vi "LSMcontroller_v59_PIzstage.vi"() -> ()   [LabVIEW 2015] (continued)
                    n4189 = call "tt_timeandsamples.vi"("bin"=w957, "refreshtime"=w951, "srateAODOtt"=w954, "tot#ofsamples"=w959) -> ("refreshrate"=w955:dbl, "refreshbuffer"=w956:i32, "timetracecycles"=w961:i32)  [unwired: 5 in]
                    n4190 = local read "bin"() -> (w958:dbl)
                    n4191 = call "2pparameters.vi"("command"="get") -> ("params out"=w970:T11)  [unwired: 1 in]
                    n4192 = Bundle By Name(cluster=w970, "Drawing Mode"=w943, "measpoints"=w959, "tt_cycles"=w961, "refreshbuffer"=w956, "refreshrate"=w955, "Vx-ref"=w962, "Vy-ref"=w964, "srate"=w953, "finite"=w966, "cont"=w965, "wavdet"=w967, "avpp"=w963, "srateAODO"=w960, "bufferAI"=w956, "bin"=w958, "Angle Img"=w950, "Vxminref"=w949, "Vxmaxref"=w948, "Vyminref"=w947, "Vymaxref"=w946, "Xpixels Img"=w945, "Ypixels Img"=w944, "Pel"=w942, "Vz-reset"=0.0, "AIoverride"=w940, "type"="Timetrace") -> (w968:T11)
                    n4193 = Reciprocal(x=w955) -> (1/x=w952:dbl)
                    n4194 = local write "refreshtime"(w952) -> ()
                    n4195 = call "2pparameters.vi"("Params in"=w968, "command"="set") -> ()  [unwired: 1 out]
                  }
                  frame "Lifetime (point)" {
                  }
                }
              }
              frame #1 {
                w973 = FALSE ("wavdet")
                n4196 = call "2pparameters.vi"("command"="get") -> ("params out"=w977:T11)  [unwired: 1 in]
                n4197 = Bundle By Name(cluster=w977, "finite"=w973, "cont"=w973, "wavdet"=TRUE) -> (w974:T11)
                n4198 = call "2pparameters.vi"("Params in"=w974, "command"="set") -> ()  [unwired: 1 out]
              }
              frame #2 {
                n4199 = local read "DO channels"() -> (w982:u16)
                n4200 = call "2pparameters.vi"("command"="get") -> ("params out"=w984:T11)  [unwired: 1 in]
                n4201 = Unbundle By Name(w984) -> ("aDO"=w983:u32[])
                n4202 = Search 1D Array(1D array=w983, element=w982) -> (index of element=w980:i32)  [unwired: 1 in]
                n4203 = Greater?(x=w980, y=-1) -> (0:w979:bool)
                n4204 = case shown="True" w979 {
                  tunnel: w980 -> [_ w993]
                  frame False {
                  }
                  frame True {
                    n4205 = local read "Meastab"() -> (w987:enum32{"X-Y Image", "Linescan", "Timetrace"})
                    n4206 = local read "Digital padding value"() -> (w988:dbl)
                    n4207 = local read "Digital time offset (s)"() -> (w989:dbl)
                    n4208 = case shown="\"Timetrace\"" w987 {
                      tunnel: [w994 w995] -> w986
                      frame "X-Y Image", Default {
                        n4209 = local read "Sampling rate"() -> (w994:dbl)
                      }
                      frame "Timetrace" {
                        n4210 = local read "srateAODOtt"() -> (w995:dbl)
                      }
                    }
                    n4211 = local read "Digital Freq (Hz)"() -> (w991:dbl)
                    n4212 = local read "Digital phase (s)"() -> (w990:dbl)
                    n4213 = local read "Digital DC (%)"() -> (w992:dbl)
                    n4214 = call "replace DO wf param.vi"("Digital Freq (Hz)"=w991, "Digital DC (%)"=w992, "Digital phase"=w990, "Sampling frequency (Hz)"=w986, "Digital time offset (s)"=w989, "index of DO wave"=w993, "padding value"=w988) -> ()  [unwired: 4 in]
                  }
                }
              }
              frame #3 {
                n4215 = case shown="True" w996 {
                  tunnel: w997 -> [_ w1004]
                  frame False {
                  }
                  frame True {
                    n4216 = local read "Meastab"() -> (w1001:enum32{"X-Y Image", "Linescan", "Timetrace"})
                    n4217 = call "waveformparamsv2.vi"("command"="get") -> ("Params out"=w1020:T15)  [unwired: 4 in, 2 out]
                    n4218 = Unbundle By Name(w1020) -> ("DO parameters"=w1019:T18)
                    n4219 = property on="refwf" class="Ring (strict)"() -> ("RingText.Text"=w1026:string)  [unwired: 2 in, 2 out]
                    n4220 = case shown="\"Timetrace\"" w1001 {
                      tunnel: [w1027 w1028] -> w1000
                      frame "X-Y Image", Default {
                        n4221 = local read "Sampling rate"() -> (w1027:dbl)
                      }
                      frame "Timetrace" {
                        n4222 = local read "srateAODOtt"() -> (w1028:dbl)
                      }
                    }
                    n4223 = call "waveformsAObuffer.vi"("command"="get") -> ("AO wf out"=w1024:waveform(dbl)[])  [unwired: 1 in]
                    n4224 = call "waveformsDObuffer.vi"("command"="get") -> ("DO wf out"=w1022:digitalwaveform[])  [unwired: 1 in]
                    n4225 = call "referfencesize.vi"("Digital waveforms in"=w1022, "Analog waveforms in"=w1024, "reference waveforms to"=w1026) -> ("number of samples"=w1017:i32)  [unwired: 2 in]
                    n4226 = Index Array(array=w1019, index=w1004) -> (element=w1018:T19)
                    n4227 = call "waveformsDObuffer.vi"("command"="get") -> ("DO wf out"=w1014:digitalwaveform[])  [unwired: 1 in]
                    n4228 = call "simple digital from wf params.vi"("waveform params"=w1018, "number of samples"=w1017) -> ("digital waveform"=w1016:digitalwaveform)
                    n4229 = property on="refwf" class="Ring (strict)"() -> ("RingText.Text"=w1006:string)  [unwired: 2 in, 2 out]
                    n4230 = Replace Array Subset(array=w1014, new element=w1016, index=w1004) -> (w1005:digitalwaveform[])
                    n4231 = call "waveformsAObuffer.vi"("command"="get") -> ("AO wf out"=w1013:waveform(dbl)[])  [unwired: 1 in]
                    n4232 = local read "wavdet"() -> (w1003:bool)
                    n4233 = call "correctwaveformsizetemp.vi"("new sampling frequency (Hz)"=w1000, "start"=FALSE, "reference waveforms to"=w1006, "Analog waveforms in"=w1013, "stop"=FALSE, "Digital waveforms in"=w1005) -> ("analog wf out"=w1009:waveform(dbl)[], "Digital wf out"=w1007:digitalwaveform[], "measpoints"=w1002:i32)
                    n4234 = local write "Analog Lines Plot"(w1009) -> ()
                    n4235 = call "GetNumCamFramesv2.vi"("Digital Waveform Graph"=w1007) -> ("Numeric"=w1008:i32)  [unwired: 10 in]
                    n4236 = local write "Digital Lines Plot"(w1007) -> ()
                    n4237 = case shown="True" w1003 {
                      tunnel: w1002 -> [_ w1029]
                      frame False {
                      }
                      frame True {
                        n4238 = local write "# of frames"(w1029) -> ()
                      }
                    }
                    n4239 = call "waveformsAObuffer.vi"("AO wf in"=w1009, "command"="set") -> ()  [unwired: 1 out]
                    n4240 = call "waveformsDObuffer.vi"("DO wf in"=w1007, "command"="set") -> ()  [unwired: 1 out]
                    n4241 = local write "Total Camera Frames"(w1008) -> ()
                  }
                }
              }
              frame #4 {
                n4242 = local read "finite samples"() -> (w1030:bool)
                n4243 = local read "continuous"() -> (w1031:bool)
                n4244 = local read "wavdet"() -> (w1032:bool)
                n4245 = call "2pparameters.vi"("command"="get") -> ("params out"=w1035:T11)  [unwired: 1 in]
                n4246 = Bundle By Name(cluster=w1035, "finite"=w1030, "cont"=w1031, "wavdet"=w1032) -> (w1033:T11)
                n4247 = call "2pparameters.vi"("Params in"=w1033, "command"="set") -> ()  [unwired: 1 out]
              }
            }
          }
          event "refwf": Value Change {
            n4248 = event-data() -> ()  [unwired: 1 in, 6 out]
            n4249 = stacked-sequence {
              frame #0 {
                n4250 = local read "Measurement"() -> (w1037:T4)
                n4251 = case shown="\"X-Y-t movie\", Default" w1037 {
                  frame "X-Y-t movie", Default {
                    n4252 = local read "avpp"() -> (w1058:i32)
                    n4253 = local read "Angle ref"() -> (w1057:dbl)
                    n4254 = local read "ROI Type"() -> (w1056:u16)
                    n4255 = local read "xpixels ref"() -> (w1053:i32)
                    n4256 = local read "Vx-min ref"() -> (w1052:dbl)
                    n4257 = local read "Vx-max ref"() -> (w1051:dbl)
                    n4258 = local read "ypixels ref"() -> (w1049:i32)
                    n4259 = local read "Vy-min ref"() -> (w1050:dbl)
                    n4260 = local read "Vy-max ref"() -> (w1046:dbl)
                    n4261 = local read "Sampling rate"() -> (w1040:dbl)
                    n4262 = local read "finite samples"() -> (w1041:bool)
                    n4263 = local read "continuous"() -> (w1044:bool)
                    n4264 = local read "wavdet"() -> (w1045:bool)
                    n4265 = local read "# of frames"() -> (w1043:i32)
                    n4266 = local read "maxbufferAI"() -> (w1042:i32)
                    n4267 = local read "Override AI buffer"() -> (w1038:bool)
                    n4268 = call "2pparameters.vi"("command"="get") -> ("params out"=w1055:T11)  [unwired: 1 in]
                    n4269 = Bundle By Name(cluster=w1055, "type"="X-Y-t movie", "avpp"=w1058, "Angle Img"=w1057, "Xpixels Img"=w1053, "Vx-min Img"=w1052, "VX-max Img"=w1051, "Ypixels Img"=w1049, "Vy-min Img"=w1050, "Vy-max Img"=w1046, "srate"=w1040, "srate Img"=w1040, "finite"=w1041, "cont"=w1044, "wavdet"=w1045, "measpoints"=w1043, "maxbufferAI"=w1042, "Drawing Mode"=w1056, "Vz-reset"=0.0, "AIoverride"=w1038) -> (w1047:T11)
                    n4270 = call "2pparameters.vi"("Params in"=w1047, "command"="set") -> ()  [unwired: 1 out]
                  }
                  frame "X-Y-Z stack" {
                    n4271 = call "2pparameters.vi"("command"="get") -> ("params out"=w1062:T11)  [unwired: 1 in]
                    n4272 = Bundle By Name(cluster=w1062, "type"="X-Y-Z stack") -> (w1060:T11)
                    n4273 = call "2pparameters.vi"("Params in"=w1060, "command"="set") -> ()  [unwired: 1 out]
                  }
                  frame "Lifetime (scan)" {
                    n4274 = call "2pparameters.vi"("command"="get") -> ("params out"=w1067:T11)  [unwired: 1 in]
                    n4275 = Bundle By Name(cluster=w1067, "type"="Lifetime (scan)") -> (w1065:T11)
                    n4276 = call "2pparameters.vi"("Params in"=w1065, "command"="set") -> ()  [unwired: 1 out]
                  }
                  frame "Lifetime (contour)" {
                    n4277 = local read "Vy-min draw"() -> (w1077:dbl)
                    n4278 = local read "Vy-max draw"() -> (w1076:dbl)
                    n4279 = local read "Vx-min draw"() -> (w1079:dbl)
                    n4280 = local read "Vx-max draw"() -> (w1078:dbl)
                    n4281 = local read "xpixels ref"() -> (w1075:i32)
                    n4282 = local read "ypixels ref"() -> (w1074:i32)
                    n4283 = local read "ROI Type"() -> (w1073:u16)
                    n4284 = local read "srateAODOtt"() -> (w1084:dbl)
                    n4285 = local read "# of frames"() -> (w1089:i32)
                    n4286 = local read "refreshtime"() -> (w1081:dbl)
                    n4287 = local read "Pel"() -> (w1072:dbl)
                    n4288 = local read "bin"() -> (w1087:dbl)
                    n4289 = local read "Override AI buffer"() -> (w1070:bool)
                    n4290 = local read "finite samples"() -> (w1096:bool)
                    n4291 = local read "srateAODOtt"() -> (w1083:dbl)
                    n4292 = local read "srateAODOtt"() -> (w1090:dbl)
                    n4293 = local read "continuous"() -> (w1095:bool)
                    n4294 = local read "Angle ref"() -> (w1080:dbl)
                    n4295 = local read "wavdet"() -> (w1097:bool)
                    n4296 = local read "Vx-ref"() -> (w1092:dbl)
                    n4297 = local read "Vy-ref"() -> (w1094:dbl)
                    n4298 = local read "avpp"() -> (w1093:i32)
                    n4299 = call "tt_timeandsamples.vi"("bin"=w1087, "refreshtime"=w1081, "srateAODOtt"=w1084, "tot#ofsamples"=w1089) -> ("refreshrate"=w1085:dbl, "refreshbuffer"=w1086:i32, "timetracecycles"=w1091:i32)  [unwired: 5 in]
                    n4300 = local read "bin"() -> (w1088:dbl)
                    n4301 = call "2pparameters.vi"("command"="get") -> ("params out"=w1100:T11)  [unwired: 1 in]
                    n4302 = Bundle By Name(cluster=w1100, "Drawing Mode"=w1073, "measpoints"=w1089, "tt_cycles"=w1091, "refreshbuffer"=w1086, "refreshrate"=w1085, "Vx-ref"=w1092, "Vy-ref"=w1094, "srate"=w1083, "finite"=w1096, "cont"=w1095, "wavdet"=w1097, "avpp"=w1093, "srateAODO"=w1090, "bufferAI"=w1086, "bin"=w1088, "Angle Img"=w1080, "Vxminref"=w1079, "Vxmaxref"=w1078, "Vyminref"=w1077, "Vymaxref"=w1076, "Xpixels Img"=w1075, "Ypixels Img"=w1074, "Pel"=w1072, "Vz-reset"=0.0, "AIoverride"=w1070, "type"="Lifetime (contour)") -> (w1098:T11)
                    n4303 = Reciprocal(x=w1085) -> (1/x=w1082:dbl)
                    n4304 = local write "refreshtime"(w1082) -> ()
                    n4305 = call "2pparameters.vi"("Params in"=w1098, "command"="set") -> ()  [unwired: 1 out]
                  }
                  frame "X-Y-Z-t movie" {
                  }
                  frame "linescan" {
                  }
                  frame "Timetrace" {
                    n4306 = local read "Vy-min draw"() -> (w1110:dbl)
                    n4307 = local read "Vy-max draw"() -> (w1109:dbl)
                    n4308 = local read "Vx-min draw"() -> (w1112:dbl)
                    n4309 = local read "Vx-max draw"() -> (w1111:dbl)
                    n4310 = local read "xpixels ref"() -> (w1108:i32)
                    n4311 = local read "ypixels ref"() -> (w1107:i32)
                    n4312 = local read "ROI Type"() -> (w1106:u16)
                    n4313 = local read "srateAODOtt"() -> (w1117:dbl)
                    n4314 = local read "# of frames"() -> (w1122:i32)
                    n4315 = local read "refreshtime"() -> (w1114:dbl)
                    n4316 = local read "Pel"() -> (w1105:dbl)
                    n4317 = local read "bin"() -> (w1120:dbl)
                    n4318 = local read "Override AI buffer"() -> (w1103:bool)
                    n4319 = local read "finite samples"() -> (w1129:bool)
                    n4320 = local read "srateAODOtt"() -> (w1116:dbl)
                    n4321 = local read "srateAODOtt"() -> (w1123:dbl)
                    n4322 = local read "continuous"() -> (w1128:bool)
                    n4323 = local read "Angle ref"() -> (w1113:dbl)
                    n4324 = local read "wavdet"() -> (w1130:bool)
                    n4325 = local read "Vx-ref"() -> (w1125:dbl)
                    n4326 = local read "Vy-ref"() -> (w1127:dbl)
                    n4327 = local read "avpp"() -> (w1126:i32)
                    n4328 = call "tt_timeandsamples.vi"("bin"=w1120, "refreshtime"=w1114, "srateAODOtt"=w1117, "tot#ofsamples"=w1122) -> ("refreshrate"=w1118:dbl, "refreshbuffer"=w1119:i32, "timetracecycles"=w1124:i32)  [unwired: 5 in]
                    n4329 = local read "bin"() -> (w1121:dbl)
                    n4330 = call "2pparameters.vi"("command"="get") -> ("params out"=w1133:T11)  [unwired: 1 in]
                    n4331 = Bundle By Name(cluster=w1133, "Drawing Mode"=w1106, "measpoints"=w1122, "tt_cycles"=w1124, "refreshbuffer"=w1119, "refreshrate"=w1118, "Vx-ref"=w1125, "Vy-ref"=w1127, "srate"=w1116, "finite"=w1129, "cont"=w1128, "wavdet"=w1130, "avpp"=w1126, "srateAODO"=w1123, "bufferAI"=w1119, "bin"=w1121, "Angle Img"=w1113, "Vxminref"=w1112, "Vxmaxref"=w1111, "Vyminref"=w1110, "Vymaxref"=w1109, "Xpixels Img"=w1108, "Ypixels Img"=w1107, "Pel"=w1105, "Vz-reset"=0.0, "AIoverride"=w1103, "type"="Timetrace") -> (w1131:T11)
                    n4332 = Reciprocal(x=w1118) -> (1/x=w1115:dbl)
                    n4333 = local write "refreshtime"(w1115) -> ()
                    n4334 = call "2pparameters.vi"("Params in"=w1131, "command"="set") -> ()  [unwired: 1 out]
                  }
                  frame "Lifetime (point)" {
                  }
                }
              }
              frame #1 {
                w1136 = FALSE ("wavdet")
                n4335 = call "2pparameters.vi"("command"="get") -> ("params out"=w1140:T11)  [unwired: 1 in]
                n4336 = Bundle By Name(cluster=w1140, "finite"=w1136, "cont"=w1136, "wavdet"=TRUE) -> (w1137:T11)
                n4337 = call "2pparameters.vi"("Params in"=w1137, "command"="set") -> ()  [unwired: 1 out]
              }
              frame #2 {
                n4338 = local read "Meastab"() -> (w1145:enum32{"X-Y Image", "Linescan", "Timetrace"})
                n4339 = property on="refwf" class="Ring (strict)"() -> ("RingText.Text"=w1148:string)  [unwired: 2 in, 2 out]
                n4340 = case shown="\"Timetrace\"" w1145 {
                  tunnel: [w1158 w1159] -> w1144
                  frame "X-Y Image", Default {
                    n4341 = local read "Sampling rate"() -> (w1158:dbl)
                  }
                  frame "Timetrace" {
                    n4342 = local read "srateAODOtt"() -> (w1159:dbl)
                  }
                }
                n4343 = call "waveformsAObuffer.vi"("command"="get") -> ("AO wf out"=w1157:waveform(dbl)[])  [unwired: 1 in]
                n4344 = local read "wavdet"() -> (w1147:bool)
                n4345 = call "waveformsDObuffer.vi"("command"="get") -> ("DO wf out"=w1153:digitalwaveform[])  [unwired: 1 in]
                n4346 = call "correctwaveformsizetemp.vi"("new sampling frequency (Hz)"=w1144, "start"=FALSE, "reference waveforms to"=w1148, "Analog waveforms in"=w1157, "stop"=FALSE, "Digital waveforms in"=w1153) -> ("analog wf out"=w1151:waveform(dbl)[], "Digital wf out"=w1149:digitalwaveform[], "measpoints"=w1146:i32)
                n4347 = local write "Analog Lines Plot"(w1151) -> ()
                n4348 = call "GetNumCamFramesv2.vi"("Digital Waveform Graph"=w1149) -> ("Numeric"=w1150:i32)  [unwired: 10 in]
                n4349 = local write "Digital Lines Plot"(w1149) -> ()
                n4350 = call "waveformsDObuffer.vi"("DO wf in"=w1149, "command"="set") -> ()  [unwired: 1 out]
                n4351 = call "waveformsAObuffer.vi"("AO wf in"=w1151, "command"="set") -> ()  [unwired: 1 out]
                n4352 = local write "Total Camera Frames"(w1150) -> ()
                n4353 = case shown="True" w1147 {
                  tunnel: w1146 -> [_ w1160]
                  frame False {
                  }
                  frame True {
                    n4354 = local write "# of frames"(w1160) -> ()
                  }
                }
              }
              frame #3 {
                n4355 = local read "finite samples"() -> (w1161:bool)
                n4356 = local read "continuous"() -> (w1162:bool)
                n4357 = local read "wavdet"() -> (w1163:bool)
                n4358 = call "2pparameters.vi"("command"="get") -> ("params out"=w1166:T11)  [unwired: 1 in]
                n4359 = Bundle By Name(cluster=w1166, "finite"=w1161, "cont"=w1162, "wavdet"=w1163) -> (w1164:T11)
                n4360 = call "2pparameters.vi"("Params in"=w1164, "command"="set") -> ()  [unwired: 1 out]
              }
            }
          }
          event "Start amplitude (V)", "Cycles", "Baseline (V)", "Step size (V)", "DC (%)", "Period (ms)", "Repeats", "Pulses", "phase shift (ms)": Value Change {
            n4361 = event-data() -> ()  [unwired: 1 in, 6 out]
            n4362 = stacked-sequence {
              seq-local: [_ _ w1274 _ _] -> [_ _ _ w1296 _]
              seq-local: [_ _ w1273 _ _] -> [_ _ _ w1295 _]
              frame #0 {
                n4363 = local read "Measurement"() -> (w1168:T4)
                n4364 = case shown="\"X-Y-t movie\", Default" w1168 {
                  frame "X-Y-t movie", Default {
                    n4365 = local read "avpp"() -> (w1189:i32)
                    n4366 = local read "Angle ref"() -> (w1188:dbl)
                    n4367 = local read "ROI Type"() -> (w1187:u16)
                    n4368 = local read "xpixels ref"() -> (w1184:i32)
                    n4369 = local read "Vx-min ref"() -> (w1183:dbl)
                    n4370 = local read "Vx-max ref"() -> (w1182:dbl)
                    n4371 = local read "ypixels ref"() -> (w1180:i32)
                    n4372 = local read "Vy-min ref"() -> (w1181:dbl)
                    n4373 = local read "Vy-max ref"() -> (w1177:dbl)
                    n4374 = local read "Sampling rate"() -> (w1171:dbl)
                    n4375 = local read "finite samples"() -> (w1172:bool)
                    n4376 = local read "continuous"() -> (w1175:bool)
                    n4377 = local read "wavdet"() -> (w1176:bool)
                    n4378 = local read "# of frames"() -> (w1174:i32)
                    n4379 = local read "maxbufferAI"() -> (w1173:i32)
                    n4380 = local read "Override AI buffer"() -> (w1169:bool)
                    n4381 = call "2pparameters.vi"("command"="get") -> ("params out"=w1186:T11)  [unwired: 1 in]
                    n4382 = Bundle By Name(cluster=w1186, "type"="X-Y-t movie", "avpp"=w1189, "Angle Img"=w1188, "Xpixels Img"=w1184, "Vx-min Img"=w1183, "VX-max Img"=w1182, "Ypixels Img"=w1180, "Vy-min Img"=w1181, "Vy-max Img"=w1177, "srate"=w1171, "srate Img"=w1171, "finite"=w1172, "cont"=w1175, "wavdet"=w1176, "measpoints"=w1174, "maxbufferAI"=w1173, "Drawing Mode"=w1187, "Vz-reset"=0.0, "AIoverride"=w1169) -> (w1178:T11)
                    n4383 = call "2pparameters.vi"("Params in"=w1178, "command"="set") -> ()  [unwired: 1 out]
                  }
                  frame "X-Y-Z stack" {
                    n4384 = call "2pparameters.vi"("command"="get") -> ("params out"=w1193:T11)  [unwired: 1 in]
                    n4385 = Bundle By Name(cluster=w1193, "type"="X-Y-Z stack") -> (w1191:T11)
                    n4386 = call "2pparameters.vi"("Params in"=w1191, "command"="set") -> ()  [unwired: 1 out]
                  }
                  frame "Lifetime (scan)" {
                    n4387 = call "2pparameters.vi"("command"="get") -> ("params out"=w1198:T11)  [unwired: 1 in]
                    n4388 = Bundle By Name(cluster=w1198, "type"="Lifetime (scan)") -> (w1196:T11)
                    n4389 = call "2pparameters.vi"("Params in"=w1196, "command"="set") -> ()  [unwired: 1 out]
                  }
                  frame "Lifetime (contour)" {
                    n4390 = local read "Vy-min draw"() -> (w1208:dbl)
                    n4391 = local read "Vy-max draw"() -> (w1207:dbl)
                    n4392 = local read "Vx-min draw"() -> (w1210:dbl)
                    n4393 = local read "Vx-max draw"() -> (w1209:dbl)
                    n4394 = local read "xpixels ref"() -> (w1206:i32)
                    n4395 = local read "ypixels ref"() -> (w1205:i32)
                    n4396 = local read "ROI Type"() -> (w1204:u16)
                    n4397 = local read "srateAODOtt"() -> (w1215:dbl)
                    n4398 = local read "# of frames"() -> (w1220:i32)
                    n4399 = local read "refreshtime"() -> (w1212:dbl)
                    n4400 = local read "Pel"() -> (w1203:dbl)
                    n4401 = local read "bin"() -> (w1218:dbl)
                    n4402 = local read "Override AI buffer"() -> (w1201:bool)
                    n4403 = local read "finite samples"() -> (w1227:bool)
                    n4404 = local read "srateAODOtt"() -> (w1214:dbl)
                    n4405 = local read "srateAODOtt"() -> (w1221:dbl)
                    n4406 = local read "continuous"() -> (w1226:bool)
                    n4407 = local read "Angle ref"() -> (w1211:dbl)
                    n4408 = local read "wavdet"() -> (w1228:bool)
                    n4409 = local read "Vx-ref"() -> (w1223:dbl)
                    n4410 = local read "Vy-ref"() -> (w1225:dbl)
                    n4411 = local read "avpp"() -> (w1224:i32)
                    n4412 = call "tt_timeandsamples.vi"("bin"=w1218, "refreshtime"=w1212, "srateAODOtt"=w1215, "tot#ofsamples"=w1220) -> ("refreshrate"=w1216:dbl, "refreshbuffer"=w1217:i32, "timetracecycles"=w1222:i32)  [unwired: 5 in]
                    n4413 = local read "bin"() -> (w1219:dbl)
                    n4414 = call "2pparameters.vi"("command"="get") -> ("params out"=w1231:T11)  [unwired: 1 in]
                    n4415 = Bundle By Name(cluster=w1231, "Drawing Mode"=w1204, "measpoints"=w1220, "tt_cycles"=w1222, "refreshbuffer"=w1217, "refreshrate"=w1216, "Vx-ref"=w1223, "Vy-ref"=w1225, "srate"=w1214, "finite"=w1227, "cont"=w1226, "wavdet"=w1228, "avpp"=w1224, "srateAODO"=w1221, "bufferAI"=w1217, "bin"=w1219, "Angle Img"=w1211, "Vxminref"=w1210, "Vxmaxref"=w1209, "Vyminref"=w1208, "Vymaxref"=w1207, "Xpixels Img"=w1206, "Ypixels Img"=w1205, "Pel"=w1203, "Vz-reset"=0.0, "AIoverride"=w1201, "type"="Lifetime (contour)") -> (w1229:T11)
                    n4416 = Reciprocal(x=w1216) -> (1/x=w1213:dbl)
                    n4417 = local write "refreshtime"(w1213) -> ()
                    n4418 = call "2pparameters.vi"("Params in"=w1229, "command"="set") -> ()  [unwired: 1 out]
                  }
                  frame "X-Y-Z-t movie" {
                  }
                  frame "linescan" {
                  }
                  frame "Timetrace" {
                    n4419 = local read "Vy-min draw"() -> (w1241:dbl)
                    n4420 = local read "Vy-max draw"() -> (w1240:dbl)
                    n4421 = local read "Vx-min draw"() -> (w1243:dbl)
                    n4422 = local read "Vx-max draw"() -> (w1242:dbl)
                    n4423 = local read "xpixels ref"() -> (w1239:i32)
                    n4424 = local read "ypixels ref"() -> (w1238:i32)
                    n4425 = local read "ROI Type"() -> (w1237:u16)
                    n4426 = local read "srateAODOtt"() -> (w1248:dbl)
                    n4427 = local read "# of frames"() -> (w1253:i32)
                    n4428 = local read "refreshtime"() -> (w1245:dbl)
                    n4429 = local read "Pel"() -> (w1236:dbl)
                    n4430 = local read "bin"() -> (w1251:dbl)
                    n4431 = local read "Override AI buffer"() -> (w1234:bool)
                    n4432 = local read "finite samples"() -> (w1260:bool)
                    n4433 = local read "srateAODOtt"() -> (w1247:dbl)
                    n4434 = local read "srateAODOtt"() -> (w1254:dbl)
                    n4435 = local read "continuous"() -> (w1259:bool)
                    n4436 = local read "Angle ref"() -> (w1244:dbl)
                    n4437 = local read "wavdet"() -> (w1261:bool)
                    n4438 = local read "Vx-ref"() -> (w1256:dbl)
                    n4439 = local read "Vy-ref"() -> (w1258:dbl)
                    n4440 = local read "avpp"() -> (w1257:i32)
                    n4441 = call "tt_timeandsamples.vi"("bin"=w1251, "refreshtime"=w1245, "srateAODOtt"=w1248, "tot#ofsamples"=w1253) -> ("refreshrate"=w1249:dbl, "refreshbuffer"=w1250:i32, "timetracecycles"=w1255:i32)  [unwired: 5 in]
                    n4442 = local read "bin"() -> (w1252:dbl)
                    n4443 = call "2pparameters.vi"("command"="get") -> ("params out"=w1264:T11)  [unwired: 1 in]
                    n4444 = Bundle By Name(cluster=w1264, "Drawing Mode"=w1237, "measpoints"=w1253, "tt_cycles"=w1255, "refreshbuffer"=w1250, "refreshrate"=w1249, "Vx-ref"=w1256, "Vy-ref"=w1258, "srate"=w1247, "finite"=w1260, "cont"=w1259, "wavdet"=w1261, "avpp"=w1257, "srateAODO"=w1254, "bufferAI"=w1250, "bin"=w1252, "Angle Img"=w1244, "Vxminref"=w1243, "Vxmaxref"=w1242, "Vyminref"=w1241, "Vymaxref"=w1240, "Xpixels Img"=w1239, "Ypixels Img"=w1238, "Pel"=w1236, "Vz-reset"=0.0, "AIoverride"=w1234, "type"="Timetrace") -> (w1262:T11)
                    n4445 = Reciprocal(x=w1249) -> (1/x=w1246:dbl)
                    n4446 = local write "refreshtime"(w1246) -> ()
                    n4447 = call "2pparameters.vi"("Params in"=w1262, "command"="set") -> ()  [unwired: 1 out]
                  }
                  frame "Lifetime (point)" {
                  }
                }
              }
              frame #1 {
                w1267 = FALSE ("wavdet")
                n4448 = call "2pparameters.vi"("command"="get") -> ("params out"=w1271:T11)  [unwired: 1 in]
                n4449 = Bundle By Name(cluster=w1271, "finite"=w1267, "cont"=w1267, "wavdet"=TRUE) -> (w1268:T11)
                n4450 = call "2pparameters.vi"("Params in"=w1268, "command"="set") -> ()  [unwired: 1 out]
              }
              frame #2 {
                n4451 = local read "AO channels"() -> (w1276:u32)
                n4452 = call "2pparameters.vi"("command"="get") -> ("params out"=w1278:T11)  [unwired: 1 in]
                n4453 = Unbundle By Name(w1278) -> ("aAO"=w1277:u32[])
                n4454 = Search 1D Array(1D array=w1277, element=w1276) -> (index of element=w1274:i32)  [unwired: 1 in]
                n4455 = Greater?(x=w1274, y=-1) -> (0:w1273:bool)
                n4456 = case shown="True" w1273 {
                  tunnel: w1274 -> [_ w1292]
                  frame False {
                  }
                  frame True {
                    n4457 = local read "Meastab"() -> (w1281:enum32{"X-Y Image", "Linescan", "Timetrace"})
                    n4458 = case shown="\"Timetrace\"" w1281 {
                      tunnel: [w1293 w1294] -> w1280
                      frame "X-Y Image", Default {
                        n4459 = local read "Sampling rate"() -> (w1293:dbl)
                      }
                      frame "Timetrace" {
                        n4460 = local read "srateAODOtt"() -> (w1294:dbl)
                      }
                    }
                    n4461 = local read "Start amplitude (V)"() -> (w1289:dbl)
                    n4462 = local read "phase shift (ms)"() -> (w1284:dbl)
                    n4463 = local read "Step size (V)"() -> (w1287:dbl)
                    n4464 = local read "Baseline (V)"() -> (w1288:dbl)
                    n4465 = local read "Period (ms)"() -> (w1285:dbl)
                    n4466 = local read "padding value"() -> (w1282:dbl)
                    n4467 = local read "Repeats"() -> (w1291:dbl)
                    n4468 = local read "Cycles"() -> (w1290:dbl)
                    n4469 = local read "DC (%)"() -> (w1286:dbl)
                    n4470 = local read "Pulses"() -> (w1283:dbl)
                    n4471 = call "replace AO square wf param.vi"("Baseline (V)"=w1288, "Start amplitude (V)"=w1289, "Cycles"=w1290, "Repeats"=w1291, "index of AO wave"=w1292, "Step size (V)"=w1287, "DC (%)"=w1286, "Sampling frequency (Hz)"=w1280, "Period (ms)"=w1285, "Cycle length (s)"=w1284, "Pulses"=w1283, "padding value"=w1282) -> ()  [unwired: 4 in]
                  }
                }
              }
              frame #3 {
                n4472 = case shown="True" w1295 {
                  tunnel: w1296 -> [_ w1304]
                  frame False {
                  }
                  frame True {
                    n4473 = call "waveformparamsv2.vi"("command"="get") -> ("Params out"=w1318:T15)  [unwired: 4 in, 2 out]
                    n4474 = Unbundle By Name(w1318) -> ("AO parameters"=w1317:T16)
                    n4475 = local read "Meastab"() -> (w1299:enum32{"X-Y Image", "Linescan", "Timetrace"})
                    n4476 = case shown="\"Timetrace\"" w1299 {
                      tunnel: [w1320 w1321] -> w1308
                      frame "X-Y Image", Default {
                        n4477 = local read "Sampling rate"() -> (w1320:dbl)
                      }
                      frame "Timetrace" {
                        n4478 = local read "srateAODOtt"() -> (w1321:dbl)
                      }
                    }
                    n4479 = Index Array(array=w1317, index=w1304) -> (element=w1306:T17)
                    n4480 = call "waveformsAObuffer.vi"("command"="get") -> ("AO wf out"=w1305:waveform(dbl)[])  [unwired: 1 in]
                    n4481 = call "generateRampedSquareWave_fromAOparameters.vi"("AO params"=w1306) -> ("Waveform"=w1303:waveform(dbl))  [unwired: 1 out]
                    n4482 = property on="refwf" class="Ring (strict)"() -> ("RingText.Text"=w1307:string)  [unwired: 2 in, 2 out]
                    n4483 = Replace Array Subset(array=w1305, new element=w1303, index=w1304) -> (w1302:waveform(dbl)[])
                    n4484 = call "waveformsDObuffer.vi"("command"="get") -> ("DO wf out"=w1313:digitalwaveform[])  [unwired: 1 in]
                    n4485 = call "correctwaveformsizetemp.vi"("new sampling frequency (Hz)"=w1308, "start"=FALSE, "reference waveforms to"=w1307, "Analog waveforms in"=w1302, "stop"=FALSE, "Digital waveforms in"=w1313) -> ("analog wf out"=w1311:waveform(dbl)[], "Digital wf out"=w1309:digitalwaveform[], "measpoints"=w1300:i32)
                    n4486 = local read "wavdet"() -> (w1301:bool)
                    n4487 = local write "Analog Lines Plot"(w1311) -> ()
                    n4488 = call "GetNumCamFramesv2.vi"("Digital Waveform Graph"=w1309) -> ("Numeric"=w1310:i32)  [unwired: 10 in]
                    n4489 = local write "Digital Lines Plot"(w1309) -> ()
                    n4490 = call "waveformsAObuffer.vi"("AO wf in"=w1311, "command"="set") -> ()  [unwired: 1 out]
                    n4491 = call "waveformsDObuffer.vi"("DO wf in"=w1309, "command"="set") -> ()  [unwired: 1 out]
                    n4492 = local write "Total Camera Frames"(w1310) -> ()
                    n4493 = case shown="True" w1301 {
                      tunnel: w1300 -> [_ w1322]
                      frame False {
                      }
                      frame True {
                        n4494 = local write "# of frames"(w1322) -> ()
                      }
                    }
                  }
                }
              }
              frame #4 {
                n4495 = local read "finite samples"() -> (w1323:bool)
                n4496 = local read "continuous"() -> (w1324:bool)
                n4497 = local read "wavdet"() -> (w1325:bool)
                n4498 = call "2pparameters.vi"("command"="get") -> ("params out"=w1328:T11)  [unwired: 1 in]
                n4499 = Bundle By Name(cluster=w1328, "finite"=w1323, "cont"=w1324, "wavdet"=w1325) -> (w1326:T11)
                n4500 = call "2pparameters.vi"("Params in"=w1326, "command"="set") -> ()  [unwired: 1 out]
              }
            }
          }
          event "Amplitude (V)", "Offset (V)", "Frequency", "Tri Repeats": Value Change {
            n4501 = event-data() -> ()  [unwired: 1 in, 6 out]
            n4502 = stacked-sequence {
              seq-local: [_ _ w1436 _ _] -> [_ _ _ w1454 _]
              seq-local: [_ _ w1435 _ _] -> [_ _ _ w1453 _]
              frame #0 {
                n4503 = local read "Measurement"() -> (w1330:T4)
                n4504 = case shown="\"X-Y-t movie\", Default" w1330 {
                  frame "X-Y-t movie", Default {
                    n4505 = local read "avpp"() -> (w1351:i32)
                    n4506 = local read "Angle ref"() -> (w1350:dbl)
                    n4507 = local read "ROI Type"() -> (w1349:u16)
                    n4508 = local read "xpixels ref"() -> (w1346:i32)
                    n4509 = local read "Vx-min ref"() -> (w1345:dbl)
                    n4510 = local read "Vx-max ref"() -> (w1344:dbl)
                    n4511 = local read "ypixels ref"() -> (w1342:i32)
                    n4512 = local read "Vy-min ref"() -> (w1343:dbl)
                    n4513 = local read "Vy-max ref"() -> (w1339:dbl)
                    n4514 = local read "Sampling rate"() -> (w1333:dbl)
                    n4515 = local read "finite samples"() -> (w1334:bool)
                    n4516 = local read "continuous"() -> (w1337:bool)
                    n4517 = local read "wavdet"() -> (w1338:bool)
                    n4518 = local read "# of frames"() -> (w1336:i32)
                    n4519 = local read "maxbufferAI"() -> (w1335:i32)
                    n4520 = local read "Override AI buffer"() -> (w1331:bool)
                    n4521 = call "2pparameters.vi"("command"="get") -> ("params out"=w1348:T11)  [unwired: 1 in]
                    n4522 = Bundle By Name(cluster=w1348, "type"="X-Y-t movie", "avpp"=w1351, "Angle Img"=w1350, "Xpixels Img"=w1346, "Vx-min Img"=w1345, "VX-max Img"=w1344, "Ypixels Img"=w1342, "Vy-min Img"=w1343, "Vy-max Img"=w1339, "srate"=w1333, "srate Img"=w1333, "finite"=w1334, "cont"=w1337, "wavdet"=w1338, "measpoints"=w1336, "maxbufferAI"=w1335, "Drawing Mode"=w1349, "Vz-reset"=0.0, "AIoverride"=w1331) -> (w1340:T11)
                    n4523 = call "2pparameters.vi"("Params in"=w1340, "command"="set") -> ()  [unwired: 1 out]
                  }
                  frame "X-Y-Z stack" {
                    n4524 = call "2pparameters.vi"("command"="get") -> ("params out"=w1355:T11)  [unwired: 1 in]
                    n4525 = Bundle By Name(cluster=w1355, "type"="X-Y-Z stack") -> (w1353:T11)
                    n4526 = call "2pparameters.vi"("Params in"=w1353, "command"="set") -> ()  [unwired: 1 out]
                  }
                  frame "Lifetime (scan)" {
                    n4527 = call "2pparameters.vi"("command"="get") -> ("params out"=w1360:T11)  [unwired: 1 in]
                    n4528 = Bundle By Name(cluster=w1360, "type"="Lifetime (scan)") -> (w1358:T11)
                    n4529 = call "2pparameters.vi"("Params in"=w1358, "command"="set") -> ()  [unwired: 1 out]
                  }
                  frame "Lifetime (contour)" {
                    n4530 = local read "Vy-min draw"() -> (w1370:dbl)
                    n4531 = local read "Vy-max draw"() -> (w1369:dbl)
                    n4532 = local read "Vx-min draw"() -> (w1372:dbl)
                    n4533 = local read "Vx-max draw"() -> (w1371:dbl)
                    n4534 = local read "xpixels ref"() -> (w1368:i32)
                    n4535 = local read "ypixels ref"() -> (w1367:i32)
                    n4536 = local read "ROI Type"() -> (w1366:u16)
                    n4537 = local read "srateAODOtt"() -> (w1377:dbl)
                    n4538 = local read "# of frames"() -> (w1382:i32)
                    n4539 = local read "refreshtime"() -> (w1374:dbl)
                    n4540 = local read "Pel"() -> (w1365:dbl)
                    n4541 = local read "bin"() -> (w1380:dbl)
                    n4542 = local read "Override AI buffer"() -> (w1363:bool)
                    n4543 = local read "finite samples"() -> (w1389:bool)
                    n4544 = local read "srateAODOtt"() -> (w1376:dbl)
                    n4545 = local read "srateAODOtt"() -> (w1383:dbl)
                    n4546 = local read "continuous"() -> (w1388:bool)
                    n4547 = local read "Angle ref"() -> (w1373:dbl)
                    n4548 = local read "wavdet"() -> (w1390:bool)
                    n4549 = local read "Vx-ref"() -> (w1385:dbl)
                    n4550 = local read "Vy-ref"() -> (w1387:dbl)
                    n4551 = local read "avpp"() -> (w1386:i32)
                    n4552 = call "tt_timeandsamples.vi"("bin"=w1380, "refreshtime"=w1374, "srateAODOtt"=w1377, "tot#ofsamples"=w1382) -> ("refreshrate"=w1378:dbl, "refreshbuffer"=w1379:i32, "timetracecycles"=w1384:i32)  [unwired: 5 in]
                    n4553 = local read "bin"() -> (w1381:dbl)
                    n4554 = call "2pparameters.vi"("command"="get") -> ("params out"=w1393:T11)  [unwired: 1 in]
                    n4555 = Bundle By Name(cluster=w1393, "Drawing Mode"=w1366, "measpoints"=w1382, "tt_cycles"=w1384, "refreshbuffer"=w1379, "refreshrate"=w1378, "Vx-ref"=w1385, "Vy-ref"=w1387, "srate"=w1376, "finite"=w1389, "cont"=w1388, "wavdet"=w1390, "avpp"=w1386, "srateAODO"=w1383, "bufferAI"=w1379, "bin"=w1381, "Angle Img"=w1373, "Vxminref"=w1372, "Vxmaxref"=w1371, "Vyminref"=w1370, "Vymaxref"=w1369, "Xpixels Img"=w1368, "Ypixels Img"=w1367, "Pel"=w1365, "Vz-reset"=0.0, "AIoverride"=w1363, "type"="Lifetime (contour)") -> (w1391:T11)
                    n4556 = Reciprocal(x=w1378) -> (1/x=w1375:dbl)
                    n4557 = local write "refreshtime"(w1375) -> ()
                    n4558 = call "2pparameters.vi"("Params in"=w1391, "command"="set") -> ()  [unwired: 1 out]
                  }
                  frame "X-Y-Z-t movie" {
                  }
                  frame "linescan" {
                  }
                  frame "Timetrace" {
                    n4559 = local read "Vy-min draw"() -> (w1403:dbl)
                    n4560 = local read "Vy-max draw"() -> (w1402:dbl)
                    n4561 = local read "Vx-min draw"() -> (w1405:dbl)
                    n4562 = local read "Vx-max draw"() -> (w1404:dbl)
                    n4563 = local read "xpixels ref"() -> (w1401:i32)
                    n4564 = local read "ypixels ref"() -> (w1400:i32)
                    n4565 = local read "ROI Type"() -> (w1399:u16)
                    n4566 = local read "srateAODOtt"() -> (w1410:dbl)
                    n4567 = local read "# of frames"() -> (w1415:i32)
                    n4568 = local read "refreshtime"() -> (w1407:dbl)
                    n4569 = local read "Pel"() -> (w1398:dbl)
                    n4570 = local read "bin"() -> (w1413:dbl)
                    n4571 = local read "Override AI buffer"() -> (w1396:bool)
                    n4572 = local read "finite samples"() -> (w1422:bool)
                    n4573 = local read "srateAODOtt"() -> (w1409:dbl)
                    n4574 = local read "srateAODOtt"() -> (w1416:dbl)
                    n4575 = local read "continuous"() -> (w1421:bool)
                    n4576 = local read "Angle ref"() -> (w1406:dbl)
                    n4577 = local read "wavdet"() -> (w1423:bool)
                    n4578 = local read "Vx-ref"() -> (w1418:dbl)
                    n4579 = local read "Vy-ref"() -> (w1420:dbl)
                    n4580 = local read "avpp"() -> (w1419:i32)
                    n4581 = call "tt_timeandsamples.vi"("bin"=w1413, "refreshtime"=w1407, "srateAODOtt"=w1410, "tot#ofsamples"=w1415) -> ("refreshrate"=w1411:dbl, "refreshbuffer"=w1412:i32, "timetracecycles"=w1417:i32)  [unwired: 5 in]
                    n4582 = local read "bin"() -> (w1414:dbl)
                    n4583 = call "2pparameters.vi"("command"="get") -> ("params out"=w1426:T11)  [unwired: 1 in]
                    n4584 = Bundle By Name(cluster=w1426, "Drawing Mode"=w1399, "measpoints"=w1415, "tt_cycles"=w1417, "refreshbuffer"=w1412, "refreshrate"=w1411, "Vx-ref"=w1418, "Vy-ref"=w1420, "srate"=w1409, "finite"=w1422, "cont"=w1421, "wavdet"=w1423, "avpp"=w1419, "srateAODO"=w1416, "bufferAI"=w1412, "bin"=w1414, "Angle Img"=w1406, "Vxminref"=w1405, "Vxmaxref"=w1404, "Vyminref"=w1403, "Vymaxref"=w1402, "Xpixels Img"=w1401, "Ypixels Img"=w1400, "Pel"=w1398, "Vz-reset"=0.0, "AIoverride"=w1396, "type"="Timetrace") -> (w1424:T11)
                    n4585 = Reciprocal(x=w1411) -> (1/x=w1408:dbl)
                    n4586 = local write "refreshtime"(w1408) -> ()
                    n4587 = call "2pparameters.vi"("Params in"=w1424, "command"="set") -> ()  [unwired: 1 out]
                  }
                  frame "Lifetime (point)" {
                  }
                }
              }
              frame #1 {
                w1429 = FALSE ("wavdet")
                n4588 = call "2pparameters.vi"("command"="get") -> ("params out"=w1433:T11)  [unwired: 1 in]
                n4589 = Bundle By Name(cluster=w1433, "finite"=w1429, "cont"=w1429, "wavdet"=TRUE) -> (w1430:T11)
                n4590 = call "2pparameters.vi"("Params in"=w1430, "command"="set") -> ()  [unwired: 1 out]
              }
              frame #2 {
                n4591 = local read "AO channels"() -> (w1438:u32)
                n4592 = call "2pparameters.vi"("command"="get") -> ("params out"=w1440:T11)  [unwired: 1 in]
                n4593 = Unbundle By Name(w1440) -> ("aAO"=w1439:u32[])
                n4594 = Search 1D Array(1D array=w1439, element=w1438) -> (index of element=w1436:i32)  [unwired: 1 in]
                n4595 = Greater?(x=w1436, y=-1) -> (0:w1435:bool)
                n4596 = case shown="True" w1435 {
                  tunnel: w1436 -> [_ w1450]
                  frame False {
                  }
                  frame True {
                    n4597 = local read "Meastab"() -> (w1443:enum32{"X-Y Image", "Linescan", "Timetrace"})
                    n4598 = local read "Tri padding value"() -> (w1444:dbl)
                    n4599 = local read "Amplitude (V)"() -> (w1448:dbl)
                    n4600 = local read "Tri Phase (s)"() -> (w1445:dbl)
                    n4601 = local read "Tri Repeats"() -> (w1446:dbl)
                    n4602 = local read "Frequency"() -> (w1447:dbl)
                    n4603 = local read "Offset (V)"() -> (w1449:dbl)
                    n4604 = case shown="\"Timetrace\"" w1443 {
                      tunnel: [w1451 w1452] -> w1442
                      frame "X-Y Image", Default {
                        n4605 = local read "Sampling rate"() -> (w1451:dbl)
                      }
                      frame "Timetrace" {
                        n4606 = local read "srateAODOtt"() -> (w1452:dbl)
                      }
                    }
                    n4607 = call "replace AO tri wf param.vi"("padding value"=w1444, "index of AO wave"=w1450, "Tri phase"=w1445, "Sampling frequency (Hz)"=w1442, "Tri Repeats"=w1446, "Frequency"=w1447, "Amplitude (V)"=w1448, "Offset (V)"=w1449) -> ()
                  }
                }
              }
              frame #3 {
                n4608 = case shown="True" w1453 {
                  tunnel: w1454 -> [_ w1463]
                  frame False {
                  }
                  frame True {
                    n4609 = call "waveformparamsv2.vi"("command"="get") -> ("Params out"=w1476:T15)  [unwired: 4 in, 2 out]
                    n4610 = Unbundle By Name(w1476) -> ("AO parameters"=w1475:T16)
                    n4611 = local read "Meastab"() -> (w1458:enum32{"X-Y Image", "Linescan", "Timetrace"})
                    n4612 = case shown="\"Timetrace\"" w1458 {
                      tunnel: [w1478 w1479] -> w1457
                      frame "X-Y Image", Default {
                        n4613 = local read "Sampling rate"() -> (w1478:dbl)
                      }
                      frame "Timetrace" {
                        n4614 = local read "srateAODOtt"() -> (w1479:dbl)
                      }
                    }
                    n4615 = Index Array(array=w1475, index=w1463) -> (element=w1465:T17)
                    n4616 = call "waveformsAObuffer.vi"("command"="get") -> ("AO wf out"=w1464:waveform(dbl)[])  [unwired: 1 in]
                    n4617 = call "generateTriWave_fromAOparameters.vi"("AO params"=w1465) -> ("Waveform"=w1462:waveform(dbl))  [unwired: 1 out]
                    n4618 = property on="refwf" class="Ring (strict)"() -> ("RingText.Text"=w1466:string)  [unwired: 2 in, 2 out]
                    n4619 = Replace Array Subset(array=w1464, new element=w1462, index=w1463) -> (w1461:waveform(dbl)[])
                    n4620 = call "waveformsDObuffer.vi"("command"="get") -> ("DO wf out"=w1471:digitalwaveform[])  [unwired: 1 in]
                    n4621 = call "correctwaveformsizetemp.vi"("new sampling frequency (Hz)"=w1457, "start"=FALSE, "reference waveforms to"=w1466, "Analog waveforms in"=w1461, "stop"=FALSE, "Digital waveforms in"=w1471) -> ("analog wf out"=w1469:waveform(dbl)[], "Digital wf out"=w1467:digitalwaveform[], "measpoints"=w1459:i32)
                    n4622 = local read "wavdet"() -> (w1460:bool)
                    n4623 = local write "Analog Lines Plot"(w1469) -> ()
                    n4624 = call "GetNumCamFramesv2.vi"("Digital Waveform Graph"=w1467) -> ("Numeric"=w1468:i32)  [unwired: 10 in]
                    n4625 = local write "Digital Lines Plot"(w1467) -> ()
                    n4626 = call "waveformsAObuffer.vi"("AO wf in"=w1469, "command"="set") -> ()  [unwired: 1 out]
                    n4627 = call "waveformsDObuffer.vi"("DO wf in"=w1467, "command"="set") -> ()  [unwired: 1 out]
                    n4628 = local write "Total Camera Frames"(w1468) -> ()
                    n4629 = case shown="True" w1460 {
                      tunnel: w1459 -> [_ w1480]
                      frame False {
                      }
                      frame True {
                        n4630 = local write "# of frames"(w1480) -> ()
                      }
                    }
                  }
                }
              }
              frame #4 {
                n4631 = local read "finite samples"() -> (w1481:bool)
                n4632 = local read "continuous"() -> (w1482:bool)
                n4633 = local read "wavdet"() -> (w1483:bool)
                n4634 = call "2pparameters.vi"("command"="get") -> ("params out"=w1486:T11)  [unwired: 1 in]
                n4635 = Bundle By Name(cluster=w1486, "finite"=w1481, "cont"=w1482, "wavdet"=w1483) -> (w1484:T11)
                n4636 = call "2pparameters.vi"("Params in"=w1484, "command"="set") -> ()  [unwired: 1 out]
              }
            }
          }
          event "Load Matlab Waveform": Value Change {
            n4637 = event-data() -> ()  [unwired: 1 in, 6 out]
            n4638 = stacked-sequence {
              seq-local: [_ _ w1594 _ _] -> [_ _ _ w1609 _]
              seq-local: [_ _ w1593 _ _] -> [_ _ _ w1608 _]
              frame #0 {
                n4639 = local read "Measurement"() -> (w1488:T4)
                n4640 = case shown="\"X-Y-t movie\", Default" w1488 {
                  frame "X-Y-t movie", Default {
                    n4641 = local read "avpp"() -> (w1509:i32)
                    n4642 = local read "Angle ref"() -> (w1508:dbl)
                    n4643 = local read "ROI Type"() -> (w1507:u16)
                    n4644 = local read "xpixels ref"() -> (w1504:i32)
                    n4645 = local read "Vx-min ref"() -> (w1503:dbl)
                    n4646 = local read "Vx-max ref"() -> (w1502:dbl)
                    n4647 = local read "ypixels ref"() -> (w1500:i32)
                    n4648 = local read "Vy-min ref"() -> (w1501:dbl)
                    n4649 = local read "Vy-max ref"() -> (w1497:dbl)
                    n4650 = local read "Sampling rate"() -> (w1491:dbl)
                    n4651 = local read "finite samples"() -> (w1492:bool)
                    n4652 = local read "continuous"() -> (w1495:bool)
                    n4653 = local read "wavdet"() -> (w1496:bool)
                    n4654 = local read "# of frames"() -> (w1494:i32)
                    n4655 = local read "maxbufferAI"() -> (w1493:i32)
                    n4656 = local read "Override AI buffer"() -> (w1489:bool)
                    n4657 = call "2pparameters.vi"("command"="get") -> ("params out"=w1506:T11)  [unwired: 1 in]
                    n4658 = Bundle By Name(cluster=w1506, "type"="X-Y-t movie", "avpp"=w1509, "Angle Img"=w1508, "Xpixels Img"=w1504, "Vx-min Img"=w1503, "VX-max Img"=w1502, "Ypixels Img"=w1500, "Vy-min Img"=w1501, "Vy-max Img"=w1497, "srate"=w1491, "srate Img"=w1491, "finite"=w1492, "cont"=w1495, "wavdet"=w1496, "measpoints"=w1494, "maxbufferAI"=w1493, "Drawing Mode"=w1507, "Vz-reset"=0.0, "AIoverride"=w1489) -> (w1498:T11)
                    n4659 = call "2pparameters.vi"("Params in"=w1498, "command"="set") -> ()  [unwired: 1 out]
                  }
                  frame "X-Y-Z stack" {
                    n4660 = call "2pparameters.vi"("command"="get") -> ("params out"=w1513:T11)  [unwired: 1 in]
                    n4661 = Bundle By Name(cluster=w1513, "type"="X-Y-Z stack") -> (w1511:T11)
                    n4662 = call "2pparameters.vi"("Params in"=w1511, "command"="set") -> ()  [unwired: 1 out]
                  }
                  frame "Lifetime (scan)" {
                    n4663 = call "2pparameters.vi"("command"="get") -> ("params out"=w1518:T11)  [unwired: 1 in]
                    n4664 = Bundle By Name(cluster=w1518, "type"="Lifetime (scan)") -> (w1516:T11)
                    n4665 = call "2pparameters.vi"("Params in"=w1516, "command"="set") -> ()  [unwired: 1 out]
                  }
                  frame "Lifetime (contour)" {
                    n4666 = local read "Vy-min draw"() -> (w1528:dbl)
                    n4667 = local read "Vy-max draw"() -> (w1527:dbl)
                    n4668 = local read "Vx-min draw"() -> (w1530:dbl)
                    n4669 = local read "Vx-max draw"() -> (w1529:dbl)
                    n4670 = local read "xpixels ref"() -> (w1526:i32)
                    n4671 = local read "ypixels ref"() -> (w1525:i32)
                    n4672 = local read "ROI Type"() -> (w1524:u16)
                    n4673 = local read "srateAODOtt"() -> (w1535:dbl)
                    n4674 = local read "# of frames"() -> (w1540:i32)
                    n4675 = local read "refreshtime"() -> (w1532:dbl)
                    n4676 = local read "Pel"() -> (w1523:dbl)
                    n4677 = local read "bin"() -> (w1538:dbl)
                    n4678 = local read "Override AI buffer"() -> (w1521:bool)
                    n4679 = local read "finite samples"() -> (w1547:bool)
                    n4680 = local read "srateAODOtt"() -> (w1534:dbl)
                    n4681 = local read "srateAODOtt"() -> (w1541:dbl)
                    n4682 = local read "continuous"() -> (w1546:bool)
                    n4683 = local read "Angle ref"() -> (w1531:dbl)
                    n4684 = local read "wavdet"() -> (w1548:bool)
                    n4685 = local read "Vx-ref"() -> (w1543:dbl)
                    n4686 = local read "Vy-ref"() -> (w1545:dbl)
                    n4687 = local read "avpp"() -> (w1544:i32)
                    n4688 = call "tt_timeandsamples.vi"("bin"=w1538, "refreshtime"=w1532, "srateAODOtt"=w1535, "tot#ofsamples"=w1540) -> ("refreshrate"=w1536:dbl, "refreshbuffer"=w1537:i32, "timetracecycles"=w1542:i32)  [unwired: 5 in]
                    n4689 = local read "bin"() -> (w1539:dbl)
                    n4690 = call "2pparameters.vi"("command"="get") -> ("params out"=w1551:T11)  [unwired: 1 in]
                    n4691 = Bundle By Name(cluster=w1551, "Drawing Mode"=w1524, "measpoints"=w1540, "tt_cycles"=w1542, "refreshbuffer"=w1537, "refreshrate"=w1536, "Vx-ref"=w1543, "Vy-ref"=w1545, "srate"=w1534, "finite"=w1547, "cont"=w1546, "wavdet"=w1548, "avpp"=w1544, "srateAODO"=w1541, "bufferAI"=w1537, "bin"=w1539, "Angle Img"=w1531, "Vxminref"=w1530, "Vxmaxref"=w1529, "Vyminref"=w1528, "Vymaxref"=w1527, "Xpixels Img"=w1526, "Ypixels Img"=w1525, "Pel"=w1523, "Vz-reset"=0.0, "AIoverride"=w1521, "type"="Lifetime (contour)") -> (w1549:T11)
                    n4692 = Reciprocal(x=w1536) -> (1/x=w1533:dbl)
                    n4693 = local write "refreshtime"(w1533) -> ()
                    n4694 = call "2pparameters.vi"("Params in"=w1549, "command"="set") -> ()  [unwired: 1 out]
                  }
                  frame "X-Y-Z-t movie" {
                  }
                  frame "linescan" {
                  }
                  frame "Timetrace" {
                    n4695 = local read "Vy-min draw"() -> (w1561:dbl)
                    n4696 = local read "Vy-max draw"() -> (w1560:dbl)
                    n4697 = local read "Vx-min draw"() -> (w1563:dbl)
                    n4698 = local read "Vx-max draw"() -> (w1562:dbl)
                    n4699 = local read "xpixels ref"() -> (w1559:i32)
                    n4700 = local read "ypixels ref"() -> (w1558:i32)
                    n4701 = local read "ROI Type"() -> (w1557:u16)
                    n4702 = local read "srateAODOtt"() -> (w1568:dbl)
                    n4703 = local read "# of frames"() -> (w1573:i32)
                    n4704 = local read "refreshtime"() -> (w1565:dbl)
                    n4705 = local read "Pel"() -> (w1556:dbl)
                    n4706 = local read "bin"() -> (w1571:dbl)
                    n4707 = local read "Override AI buffer"() -> (w1554:bool)
                    n4708 = local read "finite samples"() -> (w1580:bool)
                    n4709 = local read "srateAODOtt"() -> (w1567:dbl)
                    n4710 = local read "srateAODOtt"() -> (w1574:dbl)
                    n4711 = local read "continuous"() -> (w1579:bool)
                    n4712 = local read "Angle ref"() -> (w1564:dbl)
                    n4713 = local read "wavdet"() -> (w1581:bool)
                    n4714 = local read "Vx-ref"() -> (w1576:dbl)
                    n4715 = local read "Vy-ref"() -> (w1578:dbl)
                    n4716 = local read "avpp"() -> (w1577:i32)
                    n4717 = call "tt_timeandsamples.vi"("bin"=w1571, "refreshtime"=w1565, "srateAODOtt"=w1568, "tot#ofsamples"=w1573) -> ("refreshrate"=w1569:dbl, "refreshbuffer"=w1570:i32, "timetracecycles"=w1575:i32)  [unwired: 5 in]
                    n4718 = local read "bin"() -> (w1572:dbl)
                    n4719 = call "2pparameters.vi"("command"="get") -> ("params out"=w1584:T11)  [unwired: 1 in]
                    n4720 = Bundle By Name(cluster=w1584, "Drawing Mode"=w1557, "measpoints"=w1573, "tt_cycles"=w1575, "refreshbuffer"=w1570, "refreshrate"=w1569, "Vx-ref"=w1576, "Vy-ref"=w1578, "srate"=w1567, "finite"=w1580, "cont"=w1579, "wavdet"=w1581, "avpp"=w1577, "srateAODO"=w1574, "bufferAI"=w1570, "bin"=w1572, "Angle Img"=w1564, "Vxminref"=w1563, "Vxmaxref"=w1562, "Vyminref"=w1561, "Vymaxref"=w1560, "Xpixels Img"=w1559, "Ypixels Img"=w1558, "Pel"=w1556, "Vz-reset"=0.0, "AIoverride"=w1554, "type"="Timetrace") -> (w1582:T11)
                    n4721 = Reciprocal(x=w1569) -> (1/x=w1566:dbl)
                    n4722 = local write "refreshtime"(w1566) -> ()
                    n4723 = call "2pparameters.vi"("Params in"=w1582, "command"="set") -> ()  [unwired: 1 out]
                  }
                  frame "Lifetime (point)" {
                  }
                }
              }
              frame #1 {
                w1587 = FALSE ("wavdet")
                n4724 = call "2pparameters.vi"("command"="get") -> ("params out"=w1591:T11)  [unwired: 1 in]
                n4725 = Bundle By Name(cluster=w1591, "finite"=w1587, "cont"=w1587, "wavdet"=TRUE) -> (w1588:T11)
                n4726 = call "2pparameters.vi"("Params in"=w1588, "command"="set") -> ()  [unwired: 1 out]
              }
              frame #2 {
                n4727 = local read "AO channels"() -> (w1596:u32)
                n4728 = call "2pparameters.vi"("command"="get") -> ("params out"=w1598:T11)  [unwired: 1 in]
                n4729 = Unbundle By Name(w1598) -> ("aAO"=w1597:u32[])
                n4730 = Search 1D Array(1D array=w1597, element=w1596) -> (index of element=w1594:i32)  [unwired: 1 in]
                n4731 = Greater?(x=w1594, y=-1) -> (0:w1593:bool)
                n4732 = case shown="True" w1593 {
                  tunnel: w1594 -> [_ w1605]
                  frame False {
                  }
                  frame True {
                    n4733 = local read "Meastab"() -> (w1601:enum32{"X-Y Image", "Linescan", "Timetrace"})
                    n4734 = local read "Matlab waveform path"() -> (w1603:path)
                    n4735 = local read "Matlab padding value"() -> (w1604:dbl)
                    n4736 = case shown="\"Timetrace\"" w1601 {
                      tunnel: [w1606 w1607] -> w1600
                      frame "X-Y Image", Default {
                        n4737 = local read "Sampling rate"() -> (w1606:dbl)
                      }
                      frame "Timetrace" {
                        n4738 = local read "srateAODOtt"() -> (w1607:dbl)
                      }
                    }
                    n4739 = call "matlabwfexistsdialogue.vi"("Matlab waveform path"=w1603) -> ("mtalab waveform path out"=w1602:path)
                    n4740 = call "replace AO matlab param.vi"("Sampling frequency (Hz)"=w1600, "matlab wave file"=w1602, "index of AO wave"=w1605, "padding value"=w1604) -> ()  [unwired: 7 in]
                  }
                }
              }
              frame #3 {
                n4741 = case shown="True" w1608 {
                  tunnel: w1609 -> [_ w1616]
                  frame False {
                  }
                  frame True {
                    n4742 = local read "Meastab"() -> (w1613:enum32{"X-Y Image", "Linescan", "Timetrace"})
                    n4743 = call "waveformparamsv2.vi"("command"="get") -> ("Params out"=w1619:T15)  [unwired: 4 in, 2 out]
                    n4744 = Unbundle By Name(w1619) -> ("AO parameters"=w1618:T16)
                    n4745 = case shown="\"Timetrace\"" w1613 {
                      tunnel: [w1633 w1634] -> w1612
                      frame "X-Y Image", Default {
                        n4746 = local read "Sampling rate"() -> (w1633:dbl)
                      }
                      frame "Timetrace" {
                        n4747 = local read "srateAODOtt"() -> (w1634:dbl)
                      }
                    }
                    n4748 = Index Array(array=w1618, index=w1616) -> (element=w1617:T17)
                    n4749 = call "waveformsAObuffer.vi"("command"="get") -> ("AO wf out"=w1623:waveform(dbl)[])  [unwired: 1 in]
                    n4750 = call "matlabAOwffromparam.vi"("Cluster"=w1617) -> ("Waveform"=w1621:waveform(dbl))  [unwired: 1 out]
                    n4751 = property on="refwf" class="Ring (strict)"() -> ("RingText.Text"=w1624:string)  [unwired: 2 in, 2 out]
                    n4752 = Replace Array Subset(array=w1623, new element=w1621, index=w1616) -> (w1622:waveform(dbl)[])
                    n4753 = call "waveformsDObuffer.vi"("command"="get") -> ("DO wf out"=w1629:digitalwaveform[])  [unwired: 1 in]
                    n4754 = call "correctwaveformsizetemp.vi"("new sampling frequency (Hz)"=w1612, "start"=FALSE, "reference waveforms to"=w1624, "Analog waveforms in"=w1622, "stop"=FALSE, "Digital waveforms in"=w1629) -> ("analog wf out"=w1627:waveform(dbl)[], "Digital wf out"=w1625:digitalwaveform[], "measpoints"=w1614:i32)
                    n4755 = local read "wavdet"() -> (w1615:bool)
                    n4756 = local write "Analog Lines Plot"(w1627) -> ()
                    n4757 = call "GetNumCamFramesv2.vi"("Digital Waveform Graph"=w1625) -> ("Numeric"=w1626:i32)  [unwired: 10 in]
                    n4758 = local write "Digital Lines Plot"(w1625) -> ()
                    n4759 = call "waveformsAObuffer.vi"("AO wf in"=w1627, "command"="set") -> ()  [unwired: 1 out]
                    n4760 = call "waveformsDObuffer.vi"("DO wf in"=w1625, "command"="set") -> ()  [unwired: 1 out]
                    n4761 = local write "Total Camera Frames"(w1626) -> ()
                    n4762 = case shown="True" w1615 {
                      tunnel: w1614 -> [_ w1635]
                      frame False {
                      }
                      frame True {
                        n4763 = local write "# of frames"(w1635) -> ()
                      }
                    }
                  }
                }
              }
              frame #4 {
                n4764 = local read "finite samples"() -> (w1636:bool)
                n4765 = local read "continuous"() -> (w1637:bool)
                n4766 = local read "wavdet"() -> (w1638:bool)
                n4767 = call "2pparameters.vi"("command"="get") -> ("params out"=w1641:T11)  [unwired: 1 in]
                n4768 = Bundle By Name(cluster=w1641, "finite"=w1636, "cont"=w1637, "wavdet"=w1638) -> (w1639:T11)
